vi "checkauto.vi"(0 "G-Code Array":string[](array[string]), 1 "stateAuto in":T1, 2 "Start Auto":bool, 3 "error in (no error)":errorcluster, 4 "queue":T2) -> (7 "stateAuto out":T1, 10 "error out":errorcluster)   [LabVIEW 2017]
uses:
  libraryGcode/control/Queue/QueueCMDandPOS.ctl
  libraryGcode/control/Queue/TypeDataPOS.ctl
  libraryGcode/control/UartCmdQueueUpdate.ctl
  controls/stateAutoMode.ctl
  global/GLOBAL_STATE.vi
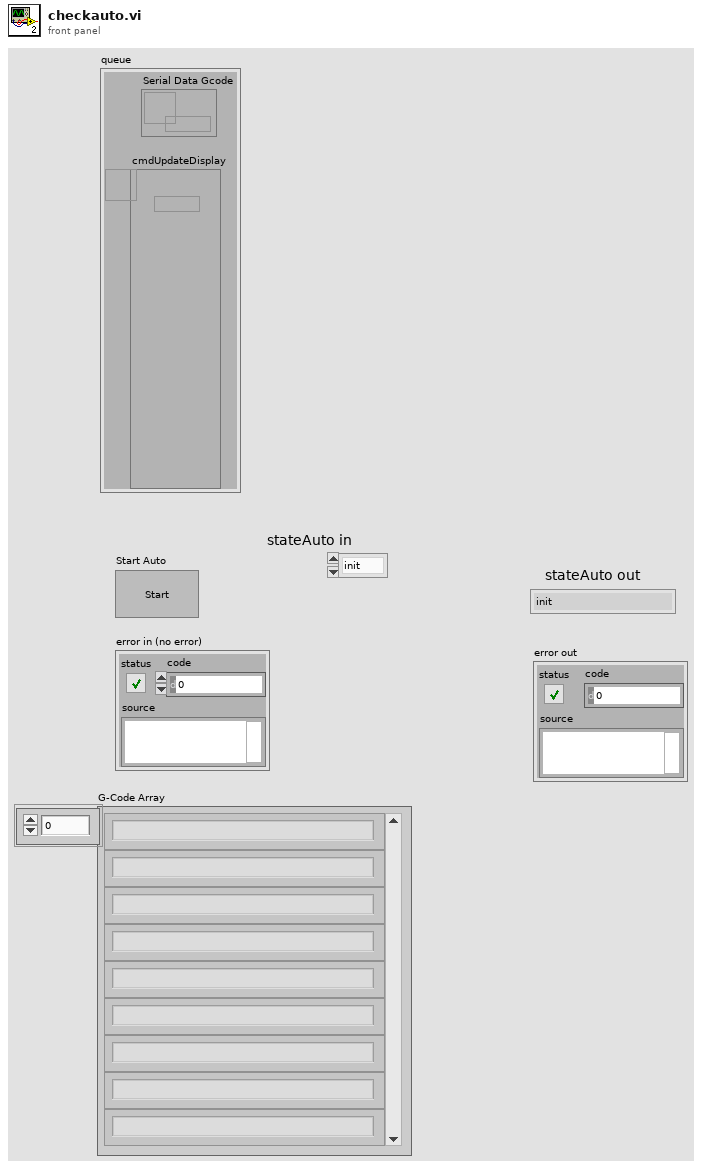
[diagram p1: front panel]
types:
  T1 = typedef "stateAutoMode.ctl" = enum16{"init", "wait", "running", "end"}
  T2 = typedef "QueueCMDandPOS.ctl" = cluster{"Serial Data Gcode":refnum<queue>, "cmdUpdateDisplay":refnum<queue>}
  T3 = typedef "UartStatusBusy.ctl" = enum16{"Running", "Waiting", "Pos", "IDLE"}
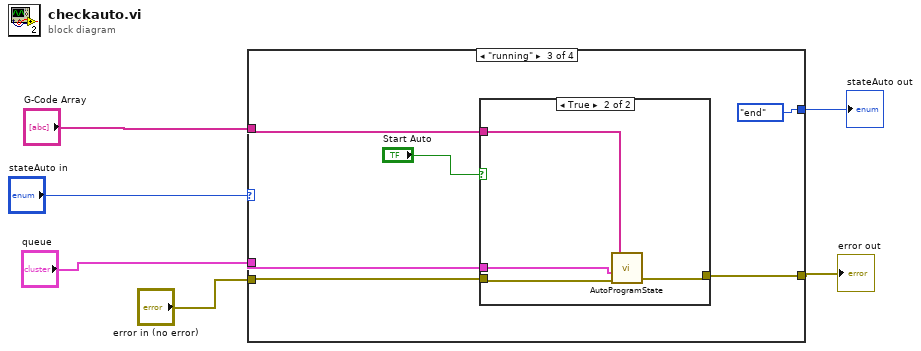
[diagram p0: block diagram]
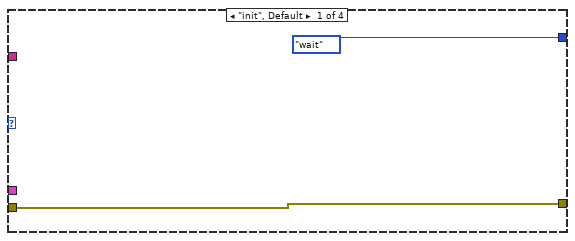
[diagram p2: hidden frame]
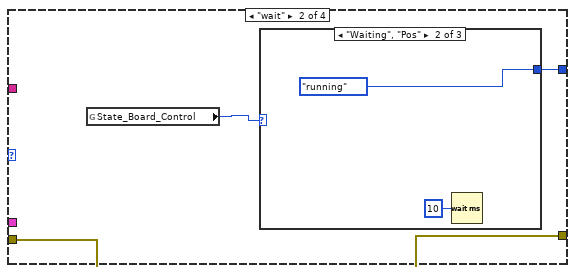
[diagram p3: hidden frame]
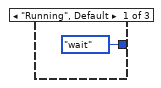
[diagram p4: hidden frame]
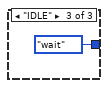
[diagram p5: hidden frame]
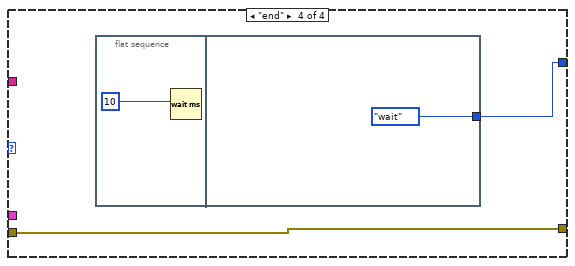
[diagram p7: hidden frame]
diagram:
  n1 = case shown="\"running\"" "stateAuto in" {
    tunnel: "error in (no error)" -> [w8 w11 w20 w28]
    tunnel: [w8 w11 w19 w28] -> w2
    tunnel: "queue" -> [_ _ w18 _]
    tunnel: "G-Code Array" -> [_ _ w17 _]
    tunnel: [stateAutoMode."wait" w10 stateAutoMode."end" w27] -> w1
    frame "init", Default {
    }
    frame "wait" {
      n2 = global read "GLOBAL_STATE.vi" "State_Board_Control"() -> (w9:T3)
      n3 = case shown="\"Waiting\", \"Pos\"" w9 {
        tunnel: [stateAutoMode."wait" stateAutoMode."running" stateAutoMode."wait"] -> w10
        frame "Running", Default {
        }
        frame "Waiting", "Pos" {
          n4 = Wait (ms)(milliseconds to wait=u32 10) -> ()  [unwired: 1 out]
        }
        frame "IDLE" {
        }
      }
    }
    frame "running" {
      n5 = case shown="True" "Start Auto" {
        tunnel: w20 -> [w22 w23]
        tunnel: w18 -> [_ w26]
        tunnel: [w22 w24] -> w19
        tunnel: w17 -> [_ w25]
        frame False {
        }
        frame True {
          n6 = call "AutoProgramState.vi"("error in (no error)"=w23, "INcluster"=w26, "G-Code Array"=w25) -> ("error in (no error) 2"=w24:errorcluster)  [unwired: 1 in, 2 out]
        }
      }
    }
    frame "end" {
      n7 = flat-sequence {
        tunnel: [stateAutoMode."wait"] -> w27
        frame #0 {
          n8 = Wait (ms)(milliseconds to wait=u32 10) -> ()  [unwired: 1 out]
        }
        frame #1 {
        }
      }
    }
  }
  "error out" <- w2
  "stateAuto out" <- w1
